vi "Connect.vi"(8 "Error In":errorcluster, 10 "Address":string, 11 "Session In":refnum<class "Session.lvclass">) -> (0 "Error Out":errorcluster, 3 "Sesssion Out":refnum<class "Session.lvclass">)   [LabVIEW 2017, in "LabSSH2.lvlib" / "Session.lvclass"]
uses:
  Session.lvclass
  Session.lvclass/Session.ctl
  <vilib>/Utility/error.llb/Error Cluster From Error Code.vi
  <vilib>/ErrorRing/Error Ring.xnode
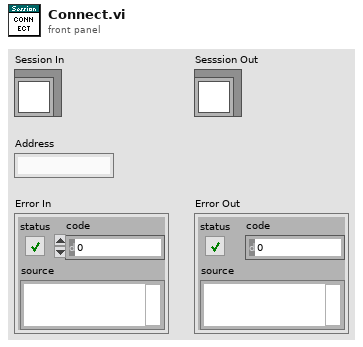
[diagram p1: front panel]
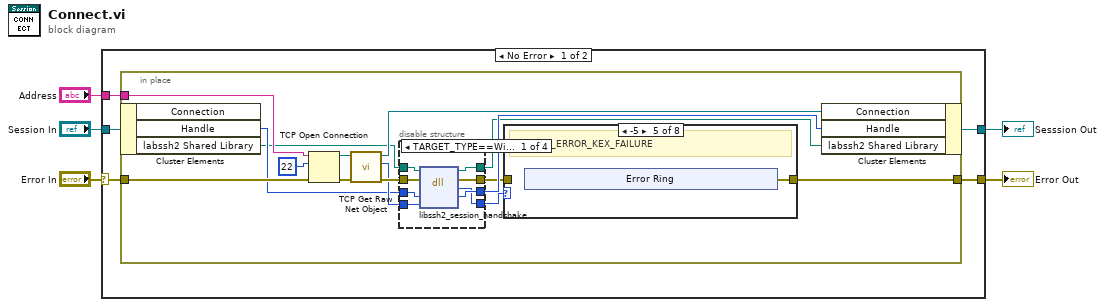
[diagram p0: block diagram]
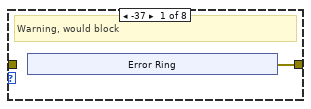
[diagram p2: hidden frame]
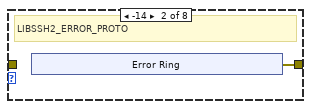
[diagram p3: hidden frame]
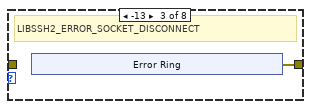
[diagram p4: hidden frame]
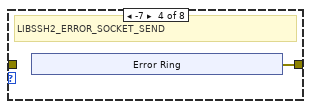
[diagram p5: hidden frame]
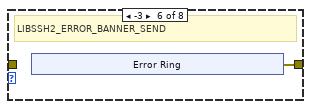
[diagram p6: hidden frame]
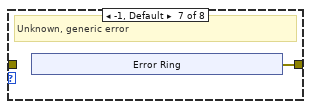
[diagram p7: hidden frame]
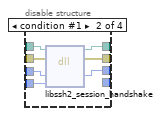
[diagram p9: hidden frame]
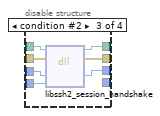
[diagram p10: hidden frame]
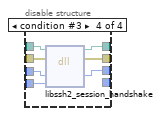
[diagram p11: hidden frame]
diagram:
  n1 = case shown="No Error" "Error In" {
    selector: "Error In" -> [w8 w92]
    tunnel: "Address" -> [w10 _]
    tunnel: [w9 w92] -> w3
    tunnel: "Session In" -> [w7 w91]
    tunnel: [w6 w91] -> w1
    frame No Error {
      n2 = in-place {
        in-place-border: w10 -> [w24]
        in-place-border: [w11] -> w9
        in-place-border: w8 -> [w23]
        n3 = in-place-cluster #1(w7) -> ("Handle"=w17:u64, "labssh2 Shared Library"=w15:path)  [unwired: 1 out]
        n4 = TCP Open Connection(address=w24, remote port or service name=u16 22, error in (no error)=w23) -> (connection ID=w21:refnum<k5>, error out=w22:errorcluster)  [unwired: 2 in]
        n5 = call <vilib>:"TCP Get Raw Net Object.vi"("error in (no error)"=w22, "connection ID"=w21) -> ("error out"=w20:errorcluster, "raw net object"=w19:u64, "connection ID out"=w18:refnum<k5>)  [unwired: 7 in]
        n6 = disable-structure shown="TARGET_TYPE==Windows, Default" {
          disable-tunnel: w15 -> [w63 w76 w81 w86]
          disable-tunnel: w20 -> [w69 w70 w77 w85]
          disable-tunnel: w17 -> [w64 w72 w82 w87]
          disable-tunnel: w19 -> [w68 w71 w83 w84]
          disable-tunnel: [w67 w75 w80 w89] -> w14
          disable-tunnel: [w66 w74 w79 w90] -> w12
          disable-tunnel: [w65 w73 w78 w88] -> w16
          disable-tunnel: [w62 _ _ _] -> w13
          frame condition #0 (active) {
            n7 = dll-call lib="D:/Users/cfield/Code/Field R&D Services/SSH/LabSSH2/LabVIEW/trunk/src/LabSSH2/Private/labssh2.*" fn="libssh2_session_handshake"(path in=w63, error in=w69, "session"=w64, "socket"=w68) -> (path out=w67:path, error out=w66:errorcluster, "result"=w62:i32, "session"=w65:u64)  [unwired: 2 in]
          }
          frame condition #1 {
            n8 = dll-call lib="D:/Users/cfield/Code/Field R&D Services/SSH/LabSSH2/LabVIEW/trunk/src/LabSSH2/Private/labssh2.*" fn="libssh2_session_handshake"(path in=w76, error in=w70, "session"=w72, "socket"=w71) -> (path out=w75:path, error out=w74:errorcluster, "session"=w73:i64)  [unwired: 3 in]
          }
          frame condition #2 {
            n9 = dll-call lib="D:/Users/cfield/Code/Field R&D Services/SSH/LabSSH2/LabVIEW/trunk/src/LabSSH2/Private/labssh2.*" fn="libssh2_session_handshake"(path in=w81, error in=w77, "session"=w82, "socket"=w83) -> (path out=w80:path, error out=w79:errorcluster, "session"=w78:u64)  [unwired: 3 in]
          }
          frame condition #3 {
            n10 = dll-call lib="D:/Users/cfield/Code/Field R&D Services/SSH/LabSSH2/LabVIEW/trunk/src/LabSSH2/Private/labssh2.*" fn="libssh2_session_handshake"(path in=w86, error in=w85, "session"=w87, "socket"=w84) -> (path out=w89:path, error out=w90:errorcluster, "session"=w88:u64)  [unwired: 3 in]
          }
        }
        n11 = case shown="-5" w13 {
          tunnel: w12 -> [_ _ _ _ _ _ _ w61]
          tunnel: [w26 w31 w36 w41 w46 w51 w56 w61] -> w11
          frame -37 {
            # "Warning, would block"
            n12 = xnode "Error Ring"() -> ("error out"=w26:errorcluster)
          }
          frame -14 {
            # "LIBSSH2_ERROR_PROTO"
            n13 = xnode "Error Ring"() -> ("error out"=w31:errorcluster)
          }
          frame -13 {
            # "LIBSSH2_ERROR_SOCKET_DISCONNECT"
            n14 = xnode "Error Ring"() -> ("error out"=w36:errorcluster)
          }
          frame -7 {
            # "LIBSSH2_ERROR_SOCKET_SEND"
            n15 = xnode "Error Ring"() -> ("error out"=w41:errorcluster)
          }
          frame -5 {
            # "LIBSSH2_ERROR_KEX_FAILURE"
            n16 = xnode "Error Ring"() -> ("error out"=w46:errorcluster)
          }
          frame -3 {
            # "LIBSSH2_ERROR_BANNER_SEND"
            n17 = xnode "Error Ring"() -> ("error out"=w51:errorcluster)
          }
          frame -1, Default {
            # "Unknown, generic error"
            n18 = xnode "Error Ring"() -> ("error out"=w56:errorcluster)
          }
          frame 0 {
            # "Success"
          }
        }
        n19 = in-place-cluster #1("Connection"=w18, "Handle"=w16, "labssh2 Shared Library"=w14) -> (w6:refnum<class "Session.lvclass">)
      }
    }
    frame Error {
    }
  }
  "Sesssion Out" <- w1
  "Error Out" <- w3
